vi "Manage Live Data.vi"(1 "New Data Point":dbl, 2 "Array":dbl[](array[numeric])) -> (0 "Updated Array":dbl[](array[numeric]))   [LabVIEW 2012]
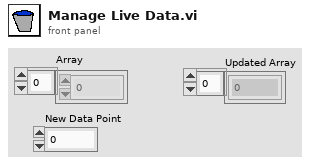
[diagram p1: front panel]
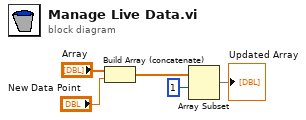
[diagram p0: block diagram]
diagram:
  n1 = Build Array (concatenate)("Array", "New Data Point") -> (w3:dbl[])
  n2 = Array Subset(array=w3, index=1) -> (→"Updated Array":dbl[])  [unwired: 1 in]
